vi "Save-characteristics.vi"(8 "error in":errorcluster, 10 "Storage element in":T1 {"Temperature characteristics"."Stand. dev. temperature" format="%#.1f"; "Temperature characteristics"."Min. temperature" format="%#.0f"; "Temperature characteristics"."Max. temperature" format="%#.0f"; "Temperature characteristics"."Average temperature" format="%#.0f"}, 11 "Storage params. ref. in":refnum<data-value>) -> (0 "error IO":errorcluster, 2 "Storage element":T1 {"Temperature characteristics"."Stand. dev. temperature" format="%#.1f"; "Temperature characteristics"."Min. temperature" format="%#.0f"; "Temperature characteristics"."Max. temperature" format="%#.0f"; "Temperature characteristics"."Average temperature" format="%#.0f"}, 3 "Storage params. ref.":refnum<data-value>)   [LabVIEW 2013, in "CameraVision.lvlib" / "CV-Main.lvclass"]
uses:
  CV-Main.lvclass
  Storage/CV-Storage.lvclass
  Buffers/Storage-buffer.ctl
  <vilib>/vision/Image Controls.llb/IMAQ Image.ctl
  Temperature/Temperature-characteristics.ctl
  Analysis/Characteristics-cluster.ctl
  Storage/CV-Storage.lvclass/CV-Storage.ctl
  Storage/Read Characteristics file reference RW.vi
  Storage/Read Save what.vi
  Storage/Read Camera suffix.vi
  Storage/Read Characteristics headers.vi
  Temperature/CV-Temperature.lvclass
  Analysis/CV-Analysis.lvclass
  Buffers/CV-Buffers.lvclass
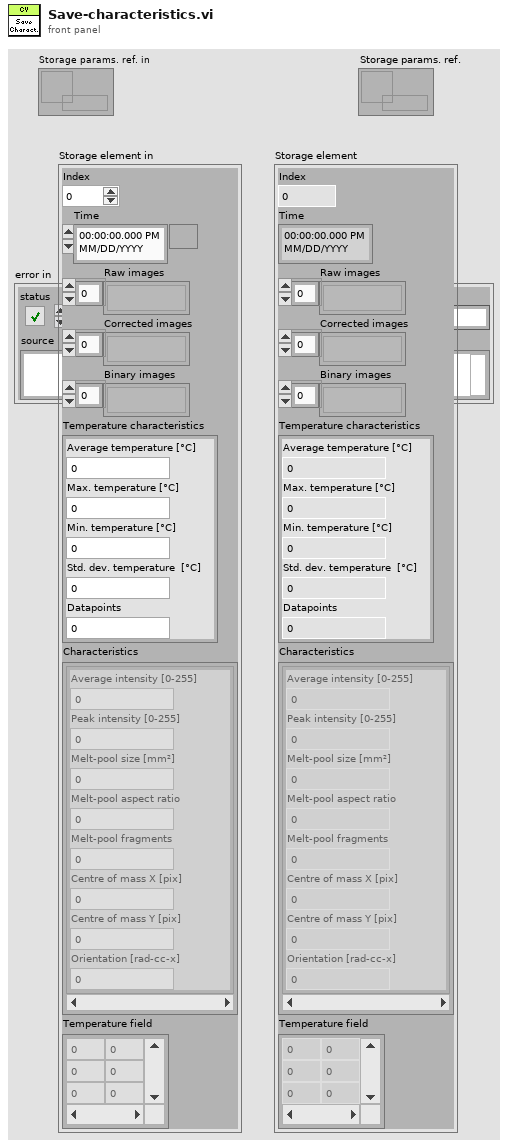
[diagram p1: front panel]
types:
  T1 = typedef "CameraVision.lvlib/CV-Buffers.lvclass/Storage-buffer.ctl" = cluster{"Index":i32, "Time":timestamp, "Raw images":T2[], "Corrected images":T2[], "Binary images":T2[], "Temperature characteristics":T3, "Characteristics":T4[], "Temperature field":dbl[][]}
  T2 = typedef "IMAQ Image.ctl" = refnum<image>
  T3 = typedef "CameraVision.lvlib/CV-Temperature.lvclass/Temperature-characteristics.ctl" = cluster{"Average temperature ":dbl, "Max. temperature":dbl, "Min. temperature":dbl, "Stand. dev. temperature":dbl, "Datapoints":dbl}
  T4 = typedef "CameraVision.lvlib/CV-Analysis.lvclass/Characteristics-cluster.ctl" = cluster{"Average intensity":dbl, "Peak intensity":dbl, "Melt-pool size":dbl, "Melt-pool aspect ratio":dbl, "Melt-pool fragments":dbl, "Centre of mass X":dbl, "Centre of mass Y":dbl, "Orientation":dbl}
  T5 = cluster{"Original":bool, "Corrected":bool, "Binary":bool, "Temperature":bool, "Characteristics":bool, "Mapping":bool, "TemperatureValues":bool}
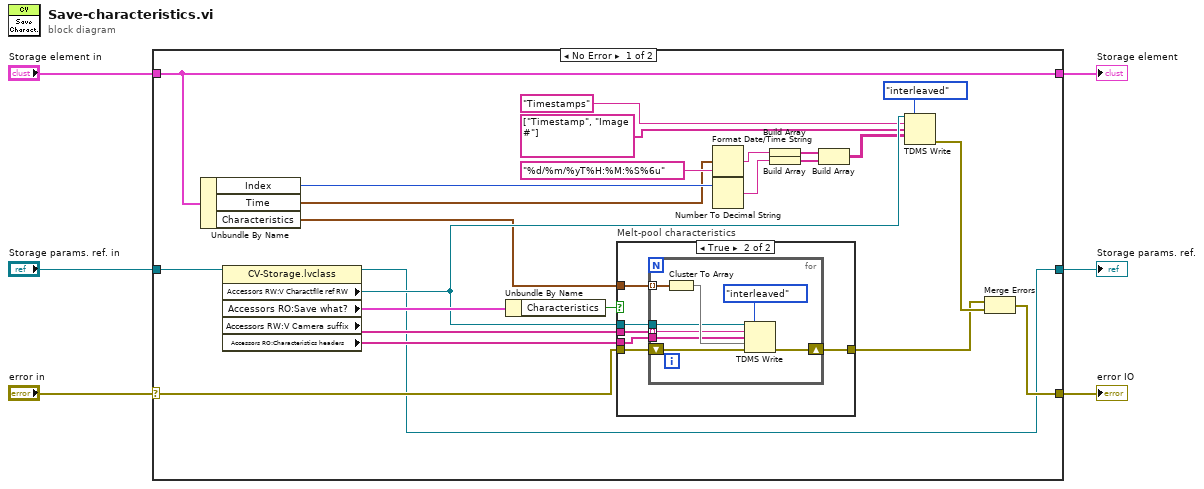
[diagram p0: block diagram]
diagram:
  n1 = case shown="No Error" "error in" {
    selector: "error in" -> [w10 w48]
    tunnel: [w9 w48] -> w6
    tunnel: "Storage params. ref. in" -> [w30 w47]
    tunnel: "Storage element in" -> [w8 w46]
    tunnel: [w7 w47] -> w2
    tunnel: [w8 w46] -> w1
    frame No Error {
      n2 = Unbundle By Name(w8) -> ("Index"=w12:i32, "Time"=w11:timestamp, "Characteristics"=w13:T4[])
      n3 = property class="CV-Storage.lvclass"(reference=w30) -> (reference out=w7:refnum<data-value>, "Accessors RW:V Charactfile ref RW"=w26:refnum<k34>, "Accessors RO:Save what?"=w27:T5, "Accessors RW:V Camera suffix"=w29:string[], "Accessors RO:Characteristics headers"=w28:string[])  [unwired: 1 in, 1 out]
      n4 = Unbundle By Name(w27) -> ("Characteristics"=w15:bool)
      n5 = case "Melt-pool characteristics" shown="True" w15 {
        tunnel: w29 -> [_ w37]
        tunnel: w26 -> [_ w36]
        tunnel: w28 -> [_ w35]
        tunnel: w10 -> [w31 w33]
        tunnel: [w31 w34] -> w14
        tunnel: w13 -> [_ w32]
        frame False {
        }
        frame True {
          n6 = for {
            tunnel: w37 -> [w44] mode=indexing
            tunnel: w35 -> [w43]
            tunnel: w36 -> [w42]
            tunnel: w32 -> [w41] mode=indexing
            shift-right: [w39] -> w34
            shift-left: w33 -> [w40]
            n7 = Cluster To Array(cluster=w41) -> (array=w45:dbl[])
            n8 = TDMS Write(0:w42, 1:enum16{"decimated", "interleaved"}."interleaved" ("data layout (0:decimated)"), 5:w44, 7:w43, 9:w45, 11:w40) -> (15:w39:errorcluster)  [unwired: 3 out]
          }
        }
      }
      n9 = Format Date/Time String(time format string (%c)="%d/%m/%yT%H:%M:%S%6u", seconds (now)=w11) -> (date/time string=w17:string)  [unwired: 1 in]
      n10 = Number To Decimal String(number=w12) -> (decimal integer string=w25:string)  [unwired: 1 in]
      n11 = Build Array(w17) -> (w21:string[])
      n12 = Build Array(w25) -> (w20:string[])
      n13 = Build Array(w21, w20) -> (w22:string[][])
      n14 = TDMS Write(0:w26, 1:enum16{"decimated", "interleaved"}."interleaved" ("data layout (0:decimated)"), 5:"Timestamps", 7:string[] ["Timestamp", "Image #"], 9:w22) -> (15:w16:errorcluster)  [unwired: 1 in, 3 out]
      n15 = Merge Errors(w14, w16) -> (w9:errorcluster)
    }
    frame Error {
    }
  }
  "error IO" <- w6
  "Storage params. ref." <- w2
  "Storage element" <- w1
